vi "Gyro_Open.vi"(0 "DIO Module":T2, 2 "Gyro Range":u8(ring) items=["250 dps"=0, "500 dps"=16, "2000 dps"=30], 3 "error in (no error)":errorcluster) -> (7 "I2CDevRef":T1 {"Device Address" format="%.0x"}, 10 "error out":errorcluster)   [LabVIEW 2011]
uses:
  <vilib>/Rock Robotics/SystemInterfaces/Typedef/FPGA_TypedefDigitalModule.ctl
  <vilib>/Rock Robotics/WPI/I2C/WPI_I2CDevRef.ctl
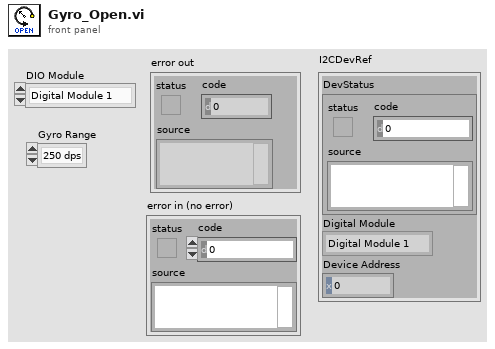
[diagram p1: front panel]
types:
  T1 = typedef "WPI_I2CDevRef.ctl" = cluster{"DevStatus":errorcluster, "Digital Module":T2, "Device Address":u8}
  T2 = typedef "FPGA_TypedefDigitalModule.ctl" = enum16{"Digital Module 1", "Digital Module 2"}
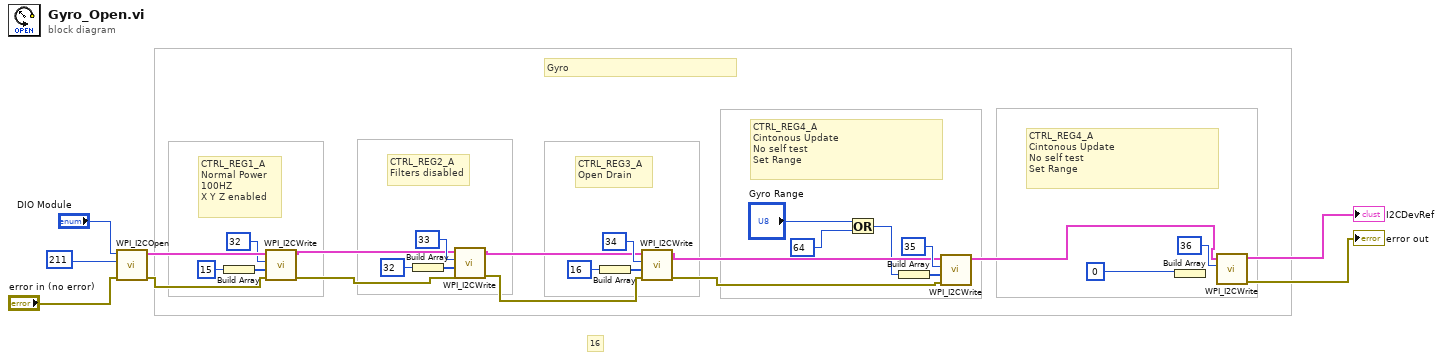
[diagram p0: block diagram]
diagram:
  # "16"
  # "CTRL_REG4_A\nCintonous Update\nNo self test\nSet Range"
  # "Gyro"
  # "CTRL_REG4_A\nCintonous Update\nNo self test\nSet Range"
  # "CTRL_REG3_A\nOpen Drain"
  # "CTRL_REG2_A\nFilters disabled"
  # "CTRL_REG1_A\nNormal Power \n100HZ\nX Y Z enabled"
  n1 = call <vilib>:"WPI_I2COpen.vi"("error in (no error)"="error in (no error)", "Device Address"=u8 211 ("Data To Send"), "Digital Module (Module 1)"="DIO Module") -> ("error out"=w13:errorcluster, "I2CDevRef"=w29:T1)  [unwired: 7 out]
  n2 = Build Array(u8 15 ("Data To Send")) -> (w26:u8[])
  n3 = call <vilib>:"WPI_I2CWrite.vi"("error in (no error)"=w13, "I2CDataToSend"=w26, "I2CRegister"=u8 32 ("Data To Send"), "I2CDevRef"=w29) -> ("error out"=w12:errorcluster, "I2CDevRef"=w21:T1)  [unwired: 1 in, 5 out]
  n4 = Build Array(u8 32 ("Data To Send")) -> (w22:u8[])
  n5 = call <vilib>:"WPI_I2CWrite.vi"("error in (no error)"=w12, "I2CDataToSend"=w22, "I2CRegister"=u8 33 ("Data To Send"), "I2CDevRef"=w21) -> ("error out"=w11:errorcluster, "I2CDevRef"=w16:T1)  [unwired: 1 in, 5 out]
  n6 = Build Array(u8 16 ("Data To Send")) -> (w18:u8[])
  n7 = call <vilib>:"WPI_I2CWrite.vi"("error in (no error)"=w11, "I2CDataToSend"=w18, "I2CRegister"=u8 34 ("Data To Send"), "I2CDevRef"=w16) -> ("error out"=w10:errorcluster, "I2CDevRef"=w15:T1)  [unwired: 1 in, 5 out]
  n8 = Or(x="Gyro Range", y=u8 64 ("Data To Send")) -> (x .or. y?=w1:u8)
  n9 = Build Array(w1) -> (w14:u8[])
  n10 = call <vilib>:"WPI_I2CWrite.vi"("error in (no error)"=w10, "I2CDataToSend"=w14, "I2CRegister"=u8 35 ("Data To Send"), "I2CDevRef"=w15) -> ("I2CDevRef"=w8:T1)  [unwired: 1 in, 6 out]
  n11 = Build Array(u8 0 ("Data To Send")) -> ()  [unwired: 1 out]
  n12 = call <vilib>:"WPI_I2CWrite.vi"("I2CRegister"=u8 36 ("Data To Send"), "I2CDevRef"=w8) -> ("error out"=→"error out":errorcluster, "I2CDevRef"=→"I2CDevRef":T1)  [unwired: 3 in, 5 out]
